vi "KGN Get Temp.vi"(8 "Fehler (Eingang, kein Fehler)":errorcluster, 9 "Info Cluster":T1, 10 "VISA-Ressourcenname":refnum<visa-resource-name>, 11 "device (Eingang)":u32) -> (0 "Fehler (Ausgang)":errorcluster, 1 "Info Cluster out":T1, 2 "VISA-Ressourcenname out":refnum<visa-resource-name>, 3 "dup device (Ausgang)":u32, 4 "Temp Cluster":T2(array[cluster]) {"humidity" format="%.2f"; "temp" format="%.2f"; "temp SP" format="%.2f"}, 6 "Kommandos gesendet":string)   [LabVIEW 2020, in "Linearisierung v2.lvlib" / "Gasteiler.lvlib" / "HovaCAL_Interface.lvlib" / "KGN.lvlib" / "KGN GUI Get.lvlib"]
uses:
  KGN GUI Get.lvlib
  Controls/Info Cluster.ctl
  get/get.lvlib
  Controls/Controls.lvlib
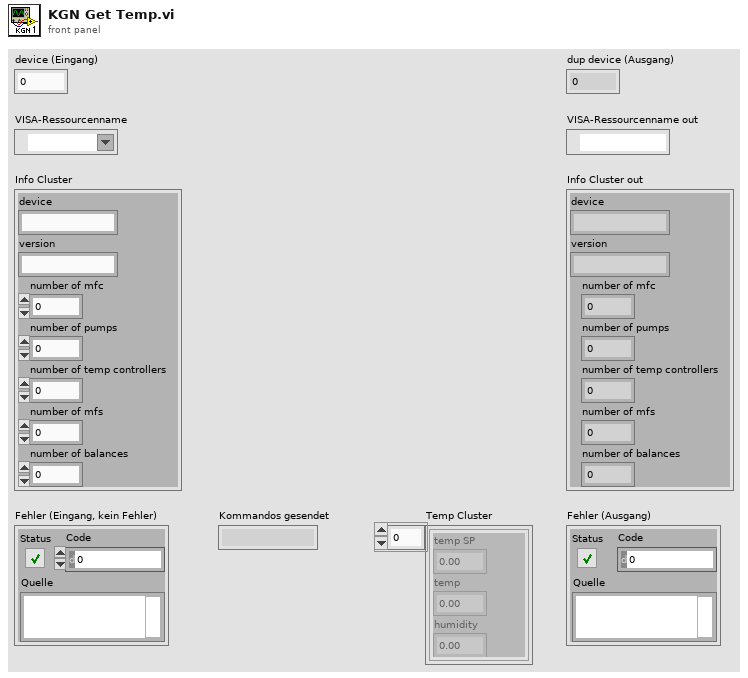
[diagram p1: front panel]
types:
  T1 = typedef "Linearisierung v2.lvlib/Gasteiler.lvlib/HovaCAL_Interface.lvlib/Controls.lvlib/Info Cluster.ctl" = cluster{"device":string, "version":string, "number of mfc":i32, "number of pumps":i32, "number of temp controllers":i32, "number of mfs":i32, "number of balances":i32}
  T2 = cluster{"temp SP":dbl, "temp":dbl, "humidity":dbl}[]
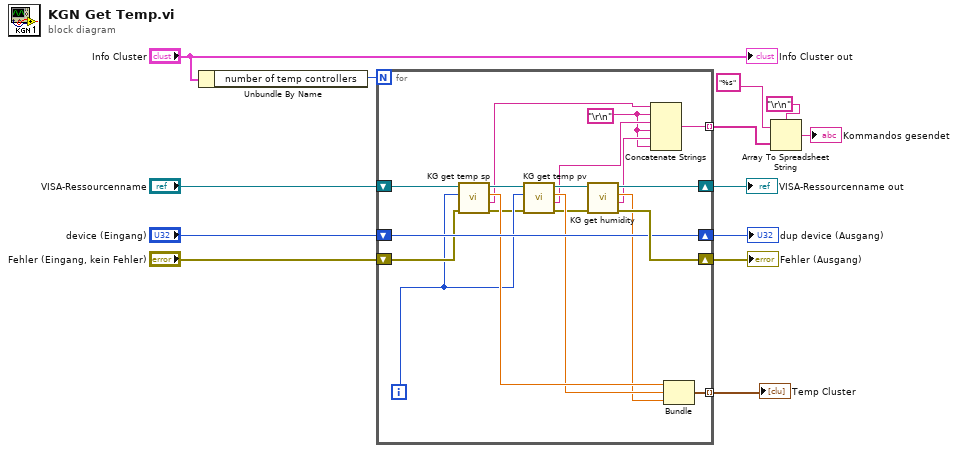
[diagram p0: block diagram]
diagram:
  n1 = Unbundle By Name("Info Cluster") -> ("number of temp controllers"=w7:i32)
  n2 = for {
    N: w7 -> [_]
    tunnel: [w26] -> w9 mode=indexing
    shift-right: [w31] -> w13
    shift-left: "device (Eingang)" -> [w31]
    shift-right: [w32] -> w12
    shift-left: "Fehler (Eingang, kein Fehler)" -> [w30]
    shift-right: [w23] -> w5
    shift-left: "VISA-Ressourcenname" -> [w24]
    tunnel: [w14] -> w2 mode=indexing
    i -> [w25]
    w15 = "\r\n"
    n3 = call "KG get temp sp.vi"("Fehler (Eingang, kein Fehler)"=w30, "controller"=w25, "VISA-Ressourcenname"=w24) -> ("Fehler (Ausgang)"=w20:errorcluster, "Kommandos gesendet"=w18:string, "temp"=w29:dbl, "VISA-Ressourcenname (Ausgang)"=w22:refnum<visa-resource-name>)  [unwired: 5 in]
    n4 = call "KG get temp pv.vi"("Fehler (Eingang, kein Fehler)"=w20, "controller"=w25, "VISA-Ressourcenname"=w22) -> ("Fehler (Ausgang)"=w19:errorcluster, "Kommando gesendet"=w17:string, "temp"=w28:dbl, "VISA-Ressourcenname (Ausgang)"=w21:refnum<visa-resource-name>)  [unwired: 5 in]
    n5 = call "KG get humidity.vi"("Fehler (Eingang, kein Fehler)"=w19, "VISA-Ressourcenname"=w21) -> ("Fehler (Ausgang)"=w32:errorcluster, "Kommandos gesendet"=w16:string, "humidity"=w27:dbl, "VISA-Ressourcenname (Ausgang)"=w23:refnum<visa-resource-name>)  [unwired: 6 in]
    n6 = Concatenate Strings(w18, w15, w17, w15, w16, w15) -> (w14:string)
    n7 = Bundle("temp"=w29, "temp"=w28, "humidity"=w27) -> (w26:cluster{"temp":dbl, "temp":dbl, "humidity":dbl})  [unwired: 1 in]
  }
  "dup device (Ausgang)" <- w13
  "Fehler (Ausgang)" <- w12
  "Temp Cluster" <- w9
  "VISA-Ressourcenname out" <- w5
  n8 = Array To Spreadsheet String(delimiter (Tab)="\r\n", array=w2, 3:"%s" ("Format-String")) -> (spreadsheet string=→"Kommandos gesendet":string)
  "Info Cluster out" <- "Info Cluster"
